vi "moveHardpointActuators.vi"(8 "error in (no error)":errorcluster, 9 "Parameters":T1, 10 "Model in":refnum<class "Model.lvclass">, 11 "ParkedMaintenanceState in":refnum<class "ParkedMaintenanceState.lvclass">) -> (0 "error out":errorcluster, 2 "Model out":refnum<class "Model.lvclass">, 3 "ParkedMaintenanceState out":refnum<class "ParkedMaintenanceState.lvclass">)   [LabVIEW 2016, in "ParkedMaintenanceState.lvclass"]
uses:
  ParkedMaintenanceState.lvclass
  DataTypes/Topics/CommandMoveHardpointActuators.ctl
  DataTypes/Topics/Parts/CommandId.ctl
  Model/Model.lvclass
  Model/Model.lvclass/Model.ctl
  ILCCommunications/ILCCommunications.lvclass/ILCCommunications.ctl
  Common_RT_HPILC/HPILC/HPILC.lvclass/HPILC.ctl
  Model/getILCCommunications.vi
  Model/setILCCommunications.vi
  ILCCommunications/getHPs.vi
  ILCCommunications/setHPs.vi
  Common_RT_HPILC/HPILC/getHPData.vi
  Common_RT_HPILC/HPILC/setHPData.vi
  DataTypes/Topics/M1M3SupportTopics.lvlib
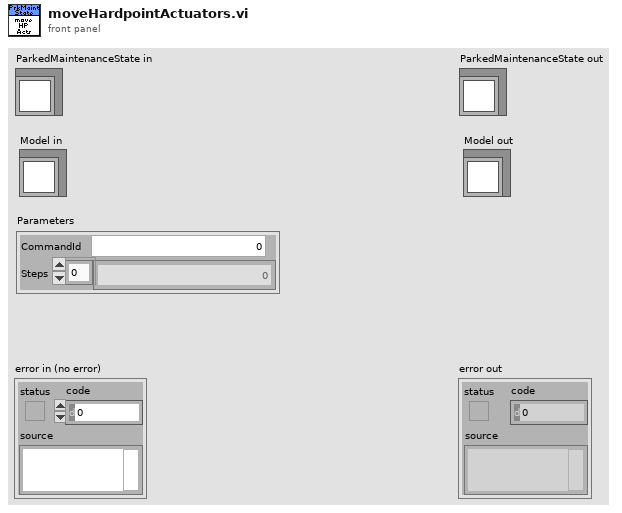
[diagram p1: front panel]
types:
  T1 = typedef "M1M3SupportTopics.lvlib/CommandMoveHardpointActuators.ctl" = cluster{"CommandId":T2, "Steps":i8[]}
  T2 = typedef "M1M3SupportTopics.lvlib/CommandId.ctl" = i32
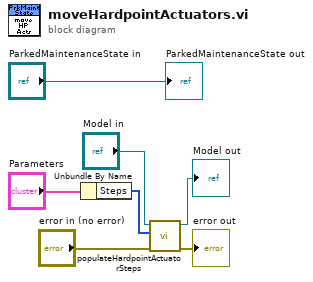
[diagram p0: block diagram]
diagram:
  n1 = Unbundle By Name("Parameters") -> ("Steps"=w5:i8[])
  n2 = call "populateHardpointActuatorSteps.vi"("error in (no error)"="error in (no error)", "Steps"=w5, "Model in"="Model in") -> ("error out"=→"error out":errorcluster, "Model out"=→"Model out":refnum<class "Model.lvclass">)  [unwired: 7 in]
  "ParkedMaintenanceState out" <- "ParkedMaintenanceState in"
